vi "CONEXAO_BT.vi"(8 "error in":errorcluster, 9 "timeout ms (60000)":i32=10000, 10 "index":i32, 11 "Endereço_Lista":string[](array[string])) -> (0 "error out":errorcluster, 3 "connection ID":refnum<k31>)   [LabVIEW 2015]
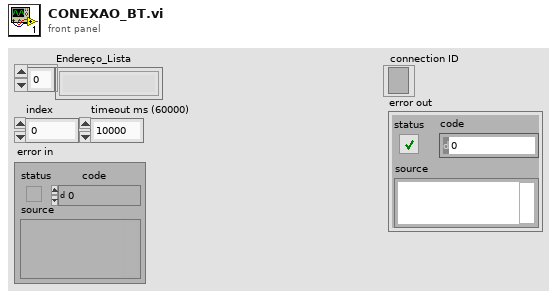
[diagram p1: front panel]
types:
  T1 = cluster{"channel":u16, "uuid":string, "service name":string, "service description":string}[]
  T2 = cluster{"channel":u16, "uuid":string, "service name":string, "service description":string}
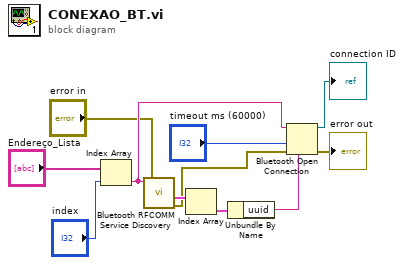
[diagram p0: block diagram]
diagram:
  n1 = Index Array(array="Endereço_Lista", index="index") -> (element=w11:string)
  n2 = call <vilib>:"Bluetooth RFCOMM Service Discovery.vi"("error in (no error)"="error in", "address in"=w11) -> ("error out"=w2:errorcluster, "service list"=w10:T1)  [unwired: 2 in, 2 out]
  n3 = Index Array(array=w10) -> (element=w9:T2)  [unwired: 1 in]
  n4 = Unbundle By Name(w9) -> ("uuid"=w8:string)
  n5 = Bluetooth Open Connection(6:w8, 8:w2, 9:"timeout ms (60000)", 11:w11) -> (0:→"error out":errorcluster, 3:→"connection ID":refnum<k31>)  [unwired: 1 in]
